vi "add-column.vi"(8 "New Column(s)":string[][](array[string]), 10 "Array In":string[][](array[string])) -> (2 "Array Out":string[][](array[string]))   [LabVIEW 2017]
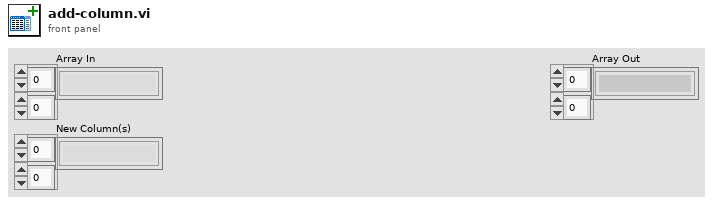
[diagram p1: front panel]
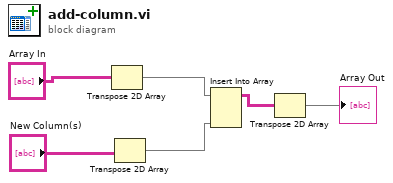
[diagram p0: block diagram]
diagram:
  n1 = Transpose 2D Array(2D array="Array In") -> (transposed array=w4:string[][])
  n2 = Transpose 2D Array(2D array="New Column(s)") -> (transposed array=w3:string[][])
  n3 = Insert Into Array(array=w4, new element=w3) -> (w2:string[][])  [unwired: 2 in]
  n4 = Transpose 2D Array(2D array=w2) -> (transposed array=→"Array Out":string[][])
